vi "GOOP_AnalyseMethodCache.vi"(7 "Actions":enum16{"Update", "ReadFromFile", "SaveToFile"}(ring), 8 "error in (no error)":errorcluster, 10 "Paths":path[](array[path]), 11 "Date And Size ID(U64)":u64[](array[numeric])) -> (0 "error out":errorcluster, 2 "PathsOut":path[](array[path]), 3 "Date And Size ID(U64)Out":u64[](array[numeric]))   [LabVIEW 2020]
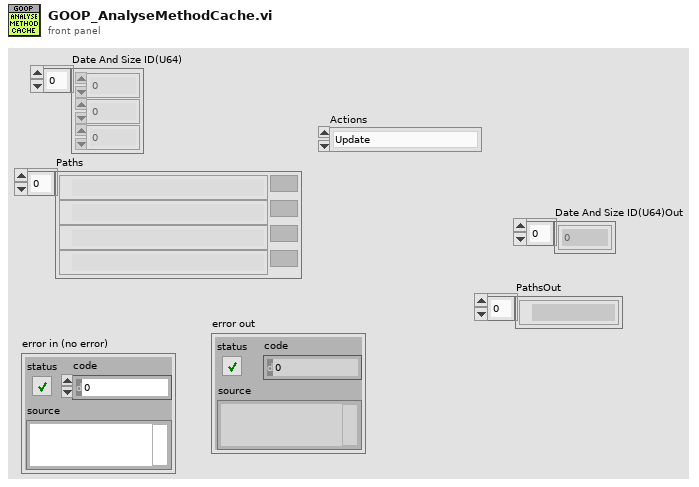
[diagram p1: front panel]
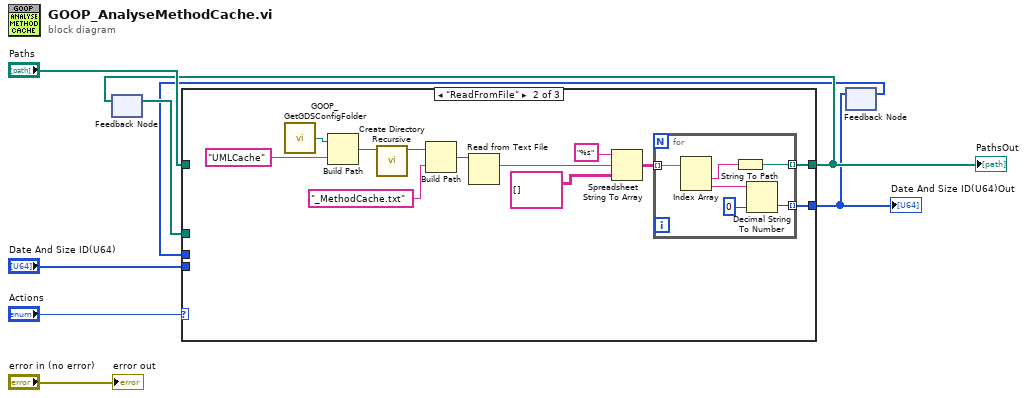
[diagram p0: block diagram]
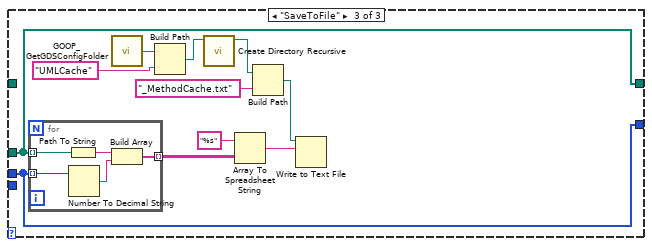
[diagram p3: hidden frame]
diagram:
  n1 = feedback #1() -> (w5:path[])  [unwired: 1 in]
  n2 = feedback #2() -> (w2:u64[])  [unwired: 1 in]
  n3 = case shown="\"ReadFromFile\"" "Actions" {
    tunnel: [w10 w12 w30] -> w6
    tunnel: "Paths" -> [w10 _ _]
    tunnel: w5 -> [_ _ w30]
    tunnel: [w9 w11 w29] -> w3
    tunnel: "Date And Size ID(U64)" -> [w9 _ _]
    tunnel: w2 -> [_ _ w29]
    frame "Update", Default {
    }
    frame "ReadFromFile" {
      n4 = call <resource>:"GOOP_GetGDSConfigFolder.vi"() -> ("GDSFolderPath"=w18:path)
      n5 = Build Path(base path=w18, name or relative path="UMLCache") -> (appended path=w15:path)
      n6 = call <vilib>:"Create Directory Recursive.vi"("directory"=w15) -> ("directory copy"=w14:path)  [unwired: 4 in, 2 out]
      n7 = Build Path(base path=w14, name or relative path="_MethodCache.txt") -> (appended path=w13:path)
      n8 = Read from Text File(file (use dialog)=w13) -> (text=w22:string)  [unwired: 3 in, 3 out]
      n9 = Spreadsheet String To Array(format string="%s", spreadsheet string=w22, array type (2D Dbl)=string[][] []) -> (array=w19:string[][])  [unwired: 1 in]
      n10 = for {
        tunnel: w19 -> [w28] mode=indexing
        tunnel: [w26] -> w12 mode=indexing
        tunnel: [w23] -> w11 mode=indexing
        n11 = Index Array(array=w28) -> (element #1=w27:string, element #2=w25:string)  [unwired: 2 in]
        n12 = String To Path(string=w27) -> (path=w26:path)
        n13 = Decimal String To Number(string=w25, default (0L)=u64 0 ("default (0 I32)")) -> (number=w23:u64)  [unwired: 1 in, 1 out]
      }
    }
    frame "SaveToFile" {
      n14 = for {
        tunnel: w30 -> [w44] mode=indexing
        tunnel: w29 -> [w42] mode=indexing
        tunnel: [w40] -> w34 mode=indexing
        n15 = Path To String(path=w44) -> (string=w43:string)
        n16 = Number To Decimal String(number=w42) -> (decimal integer string=w41:string)  [unwired: 1 in]
        n17 = Build Array(w43, w41) -> (w40:string[])
      }
      n18 = call <resource>:"GOOP_GetGDSConfigFolder.vi"() -> ("GDSFolderPath"=w39:path)
      n19 = Build Path(base path=w39, name or relative path="UMLCache") -> (appended path=w36:path)
      n20 = call <vilib>:"Create Directory Recursive.vi"("directory"=w36) -> ("directory copy"=w35:path)  [unwired: 4 in, 2 out]
      n21 = Array To Spreadsheet String(array=w34, 3:"%s" ("format string")) -> (spreadsheet string=w32:string)  [unwired: 1 in]
      n22 = Build Path(base path=w35, name or relative path="_MethodCache.txt") -> (appended path=w31:path)
      n23 = Write to Text File(file (use dialog)=w31, text=w32) -> ()  [unwired: 2 in, 3 out]
    }
  }
  "PathsOut" <- w6
  "Date And Size ID(U64)Out" <- w3
  n24 = feedback-in #1(w6) -> ()
  n25 = feedback-in #2(w3) -> ()
  "error out" <- "error in (no error)"
